vi "Destroy User Events.vi"(8 "error in":errorcluster, 11 "Master Controller in":refnum<class "EMS User Interface.lvclass">) -> (0 "error out":errorcluster, 3 "Master Controller out":refnum<class "EMS User Interface.lvclass">)   [LabVIEW 2018, in "EMS User Interface Actor.lvlib" / "EMS User Interface.lvclass"]
uses:
  EMS User Interface.lvclass
  EMS User Interface.lvclass/EMS User Interface.ctl
  EMS Generic Actor/EMS Generic/EMS Generic.lvclass
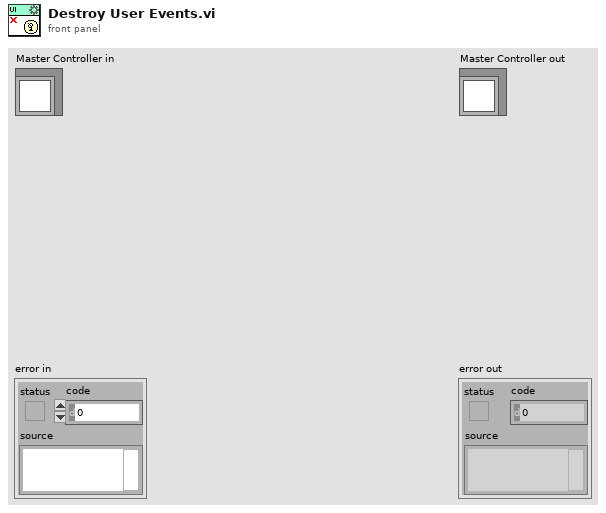
[diagram p1: front panel]
types:
  T1 = typedef "EMS User Interface Actor.lvlib/EMS User Interface.lvclass/Master Controller User Events.ctl" = cluster{"Current State":refnum<user-event>, "Current Status":refnum<user-event>, "Device List":refnum<user-event>, "P Meas":refnum<user-event>, "Q Meas":refnum<user-event>, "P Set Max":refnum<user-event>, "Q Set Max":refnum<user-event>, "IED_Status":refnum<user-event>, "Device State Information":refnum<user-event>}
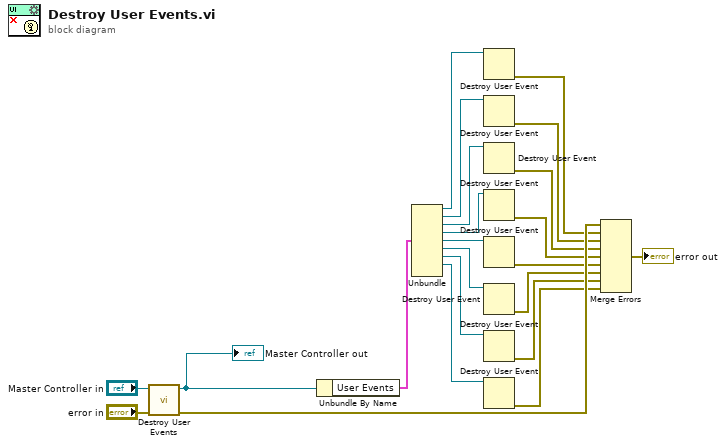
[diagram p0: block diagram]
diagram:
  n1 = call-parent "Destroy User Events.vi"("error in"="error in", "EMS Generic in"="Master Controller in") -> ("error out"=w22:errorcluster, "EMS Generic out"=w12:refnum<class "EMS User Interface.lvclass">)  [unwired: 8 in]
  "Master Controller out" <- w12
  n2 = Unbundle By Name(w12) -> ("User Events"=w20:T1)
  n3 = Unbundle(w20) -> ("Current State"=w17:refnum<user-event>, "Current Status"=w18:refnum<user-event>, "Device List"=w19:refnum<user-event>, "P Meas"=w10:refnum<user-event>, "Q Meas"=w9:refnum<user-event>, "P Set Max"=w8:refnum<user-event>, "Q Set Max"=w7:refnum<user-event>, "IED_Status"=w6:refnum<user-event>)  [unwired: 1 out]
  n4 = Destroy User Event(user event=w17) -> (error out=w16:errorcluster)  [unwired: 1 in]
  n5 = Destroy User Event(user event=w18) -> (error out=w15:errorcluster)  [unwired: 1 in]
  n6 = Destroy User Event(user event=w19) -> (error out=w14:errorcluster)  [unwired: 1 in]
  n7 = Destroy User Event(user event=w10) -> (error out=w5:errorcluster)  [unwired: 1 in]
  n8 = Destroy User Event(user event=w9) -> (error out=w4:errorcluster)  [unwired: 1 in]
  n9 = Destroy User Event(user event=w8) -> (error out=w3:errorcluster)  [unwired: 1 in]
  n10 = Destroy User Event(user event=w7) -> (error out=w2:errorcluster)  [unwired: 1 in]
  n11 = Destroy User Event(user event=w6) -> (error out=w1:errorcluster)  [unwired: 1 in]
  n12 = Merge Errors(w22, w16, w15, w14, w5, w4, w3, w2, w1) -> (→"error out":errorcluster)
